vi "TimeInterpPose2d_GetSample.vi"(9 "TimeStamp":dbl, 11 "TimeInterpPose":T1 {"Pose"."ROTATION"."SIN" format="%13.4f"; "Pose"."ROTATION"."COS" format="%13.4f"; "Pose"."ROTATION"."VALUE" format="%13.4f"; "Pose"."TRANSLATION"."Y" format="%14.3f"; "Pose"."TRANSLATION"."X" format="%14.3f"}) -> (1 "IsPresent":bool, 3 "OutputPose":T2={"TRANSLATION"={"X"=0.0, "Y"=0.0}, "ROTATION"={"VALUE"=0.0, "COS"=1.0, "SIN"=0.0}} {"ROTATION"."SIN" format="%13.4f"; "ROTATION"."COS" format="%13.4f"; "ROTATION"."VALUE" format="%13.4f"; "TRANSLATION"."Y" format="%14.3f"; "TRANSLATION"."X" format="%14.3f"})   [LabVIEW 2019, in "Trajectory_Library.lvlib"]
doc: "Calculate the output Y value for the provided X. This is done by interpolating through an array of X and Y pairs. The pairs must be ordered in increasing X value.\n\nInputs:\n - Function_Generator -- function generator data structure\n - Input Value -- The input value. \n\nOutputs:\n - Output Value -- Output value calcuated from the input value."
uses:
  Trajectory_Library.lvlib
  POSE2D.ctl
  TRANSLATION2D.ctl
  ROTATION2D.ctl
  TIME_INTERPOLATABLE_POSE.ctl
  Twist2d_GetAll.vi
  Twist2d_Create.vi
  Pose2d_Log.vi
  Pose2d_Exp.vi
  <vilib>/gmath/NI_Gmath.lvlib
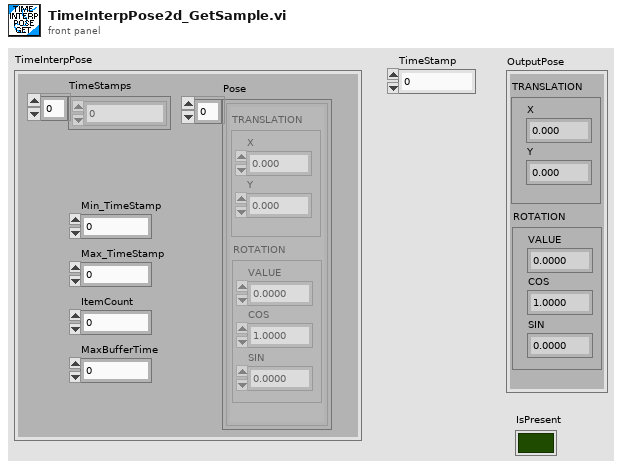
[diagram p1: front panel]
types:
  T1 = typedef "Trajectory_Library.lvlib/TIME_INTERPOLATABLE_POSE.ctl" = cluster{"TimeStamps":dbl[], "Pose":T2[], "Min_TimeStamp":dbl, "Max_TimeStamp":dbl, "ItemCount":i32, "MaxBufferTime":dbl}
  T2 = typedef "Trajectory_Library.lvlib/POSE2D.ctl" = cluster{"TRANSLATION":T3, "ROTATION":T4}
  T3 = typedef "Trajectory_Library.lvlib/TRANSLATION2D.ctl" = cluster{"X":dbl, "Y":dbl}
  T4 = typedef "Trajectory_Library.lvlib/ROTATION2D.ctl" = cluster{"VALUE":dbl, "COS":dbl, "SIN":dbl}
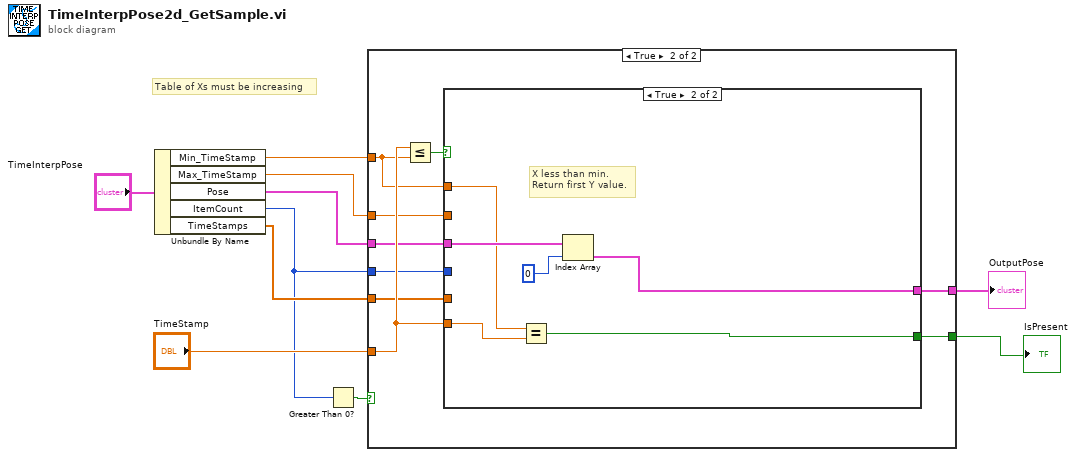
[diagram p0: block diagram]
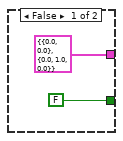
[diagram p2: hidden frame]
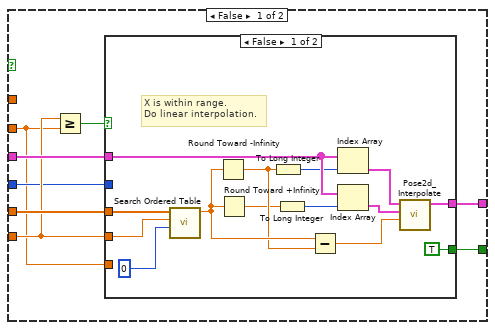
[diagram p3: hidden frame]
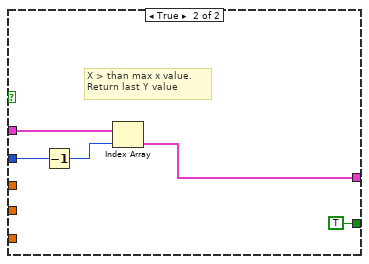
[diagram p4: hidden frame]
diagram:
  # "Table of Xs must be increasing"
  n1 = Unbundle By Name("TimeInterpPose") -> ("Min_TimeStamp"=w7:dbl, "Max_TimeStamp"=w6:dbl, "Pose"=w4:T2[], "ItemCount"=w2:i32, "TimeStamps"=w5:dbl[])
  n2 = Greater Than 0?(x=w2) -> (x > 0?=w3:bool)
  n3 = case shown="True" w3 {
    tunnel: "TimeStamp" -> [_ w20]
    tunnel: [T2 {"TRANSLATION"={"X"=0.0, "Y"=0.0}, "ROTATION"={"VALUE"=0.0, "COS"=1.0, "SIN"=0.0}} ("Table Y") w19] -> w9
    tunnel: w7 -> [_ w14]
    tunnel: w6 -> [_ w18]
    tunnel: w2 -> [_ w17]
    tunnel: w5 -> [_ w16]
    tunnel: w4 -> [_ w15]
    tunnel: [FALSE w13] -> w1
    frame False {
    }
    frame True {
      n4 = Less Or Equal?(x=w20, y=w14) -> (x <= y?=w21:bool)
      n5 = case shown="True" w21 {
        tunnel: w15 -> [w28 w54]
        tunnel: [w27 w52] -> w19
        tunnel: w20 -> [w25 w51]
        tunnel: w18 -> [w23 _]
        tunnel: w16 -> [w26 _]
        tunnel: w17 -> [w24 _]
        tunnel: w14 -> [_ w50]
        tunnel: [w22 w49] -> w13
        frame False {
          n6 = Greater Or Equal?(x=w25, y=w23) -> (x >= y?=w29:bool)
          n7 = case shown="False" w29 {
            tunnel: w28 -> [w39 w48]
            tunnel: [w40 w47] -> w27
            tunnel: w26 -> [w42 _]
            tunnel: w25 -> [w41 _]
            tunnel: w24 -> [_ w46]
            tunnel: w23 -> [_ _]
            tunnel: [TRUE TRUE] -> w22
            frame False {
              # "X is within range.  \nDo linear interpolation."
              n8 = call <vilib>:"Search Ordered Table.vi"("starting index"=0, "x value"=w41, "ordered x array"=w42) -> ("fractional index"=w34:dbl)  [unwired: 8 in]
              n9 = Round Toward -Infinity(1:w34) -> (0:w32:dbl)
              n10 = Round Toward +Infinity(x=w34) -> (ceil(x): smallest int >= x=w31:dbl)
              n11 = To Long Integer(number=w32) -> (32bit integer=w36:i32)
              n12 = To Long Integer(number=w31) -> (32bit integer=w35:i32)
              n13 = Subtract(x=w34, y=w32) -> (x-y=w33:dbl)
              n14 = Index Array(array=w39, index=w36) -> (element=w38:T2)
              n15 = Index Array(array=w39, index=w35) -> (element=w37:T2)
              n16 = call "Pose2d_Interpolate.vi"("T"=w33, "EndValue Pose"=w37, "in POSE"=w38) -> ("Interpolated Pose"=w40:T2)  [unwired: 8 in]
            }
            frame True {
              # "X > than max x value.   \nReturn last Y value"
              n17 = Decrement(x=w46) -> (x-1=w45:i32)
              n18 = Index Array(array=w48, index=w45) -> (element=w47:T2)
            }
          }
        }
        frame True {
          # "X less than min.   \nReturn first Y value."
          n19 = Equal?(x=w50, y=w51) -> (x = y?=w49:bool)
          n20 = Index Array(array=w54, index=0) -> (element=w52:T2)
        }
      }
    }
  }
  "OutputPose" <- w9
  "IsPresent" <- w1
